vi "Graph Popup.vi"(11 "Queue for data":refnum<queue>) -> ()   [LabVIEW 2019]
panel:
  out "Waveform Chart":dbl[](graph)
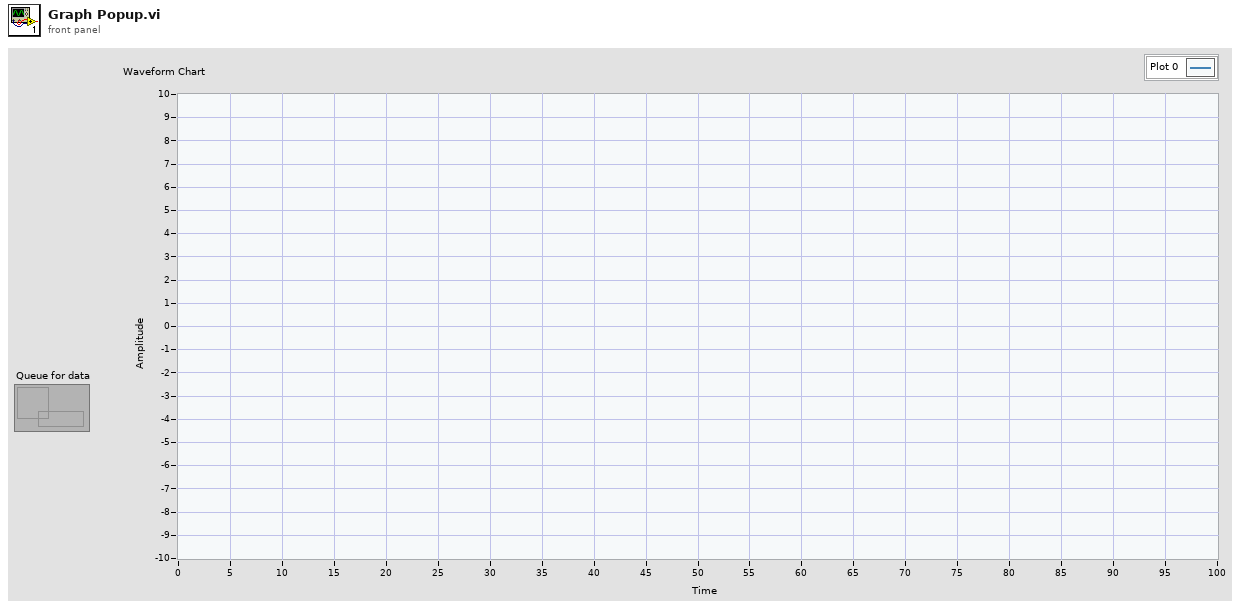
[diagram p1: front panel]
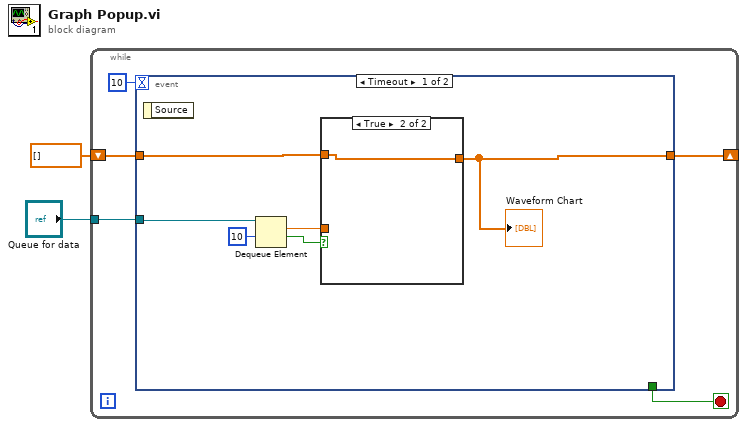
[diagram p0: block diagram]
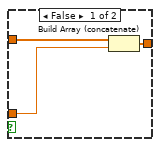
[diagram p2: hidden frame]
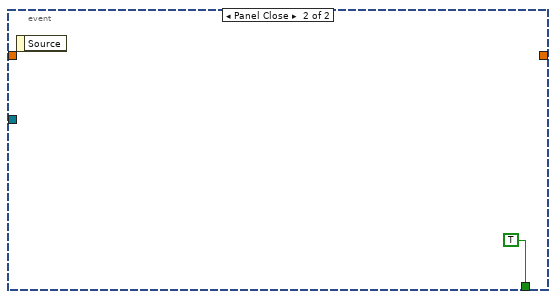
[diagram p3: hidden frame]
diagram:
  n1 = while {
    tunnel: "Queue for data" -> [w6]
    shift-right: [w4] -> _
    shift-left: dbl[] [] -> [w3]
    stop <- w7 stop-if-true
    n2 = event shown="[0] Timeout" {
      selector: _ -> [_ _]
      dyn-events: _ -> [_ _]
      timeout: 10 -> [_ _]
      tunnel: [_ TRUE] -> w7
      tunnel: w6 -> [w13 _]
      tunnel: [w9 _] -> w4
      tunnel: w3 -> [w10 _]
      event Timeout {
        n3 = event-data() -> ()  [unwired: 1 in, 1 out]
        n4 = Dequeue Element(queue=w13, timeout in ms (-1)=10) -> (element=w11:dbl, timed out?=w8:bool)  [unwired: 1 in, 2 out]
        n5 = case shown="True" w8 {
          tunnel: w11 -> [w16 _]
          tunnel: w10 -> [w15 w17]
          tunnel: [w14 w17] -> w9
          frame False {
            n6 = Build Array (concatenate)(w15, w16) -> (w14:dbl[])
          }
          frame True {
          }
        }
        "Waveform Chart" <- w9
      }
      event Panel Close {
        n7 = event-data() -> ()  [unwired: 1 in, 1 out]
      }
    }
  }
